vi "GetValue.vi"(8 "error in":errorcluster, 11 "CustomElement in":refnum<class "CustomElement.lvclass">) -> (0 "error out":errorcluster, 2 "Value":string, 3 "CustomElement out":refnum<class "CustomElement.lvclass">)   [LabVIEW 2021, in "ProligentXMLGenerator.lvlib" / "CustomElement.lvclass"]
doc: "This value need to be formated as a valid XML element."
uses:
  CustomElement.lvclass
  CustomElement.lvclass/CustomElement.ctl
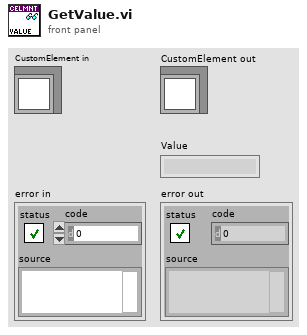
[diagram p1: front panel]
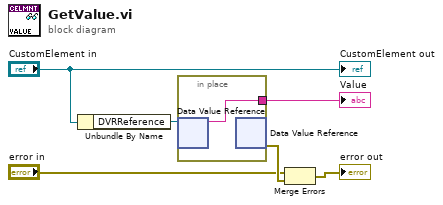
[diagram p0: block diagram]
diagram:
  n1 = Unbundle By Name("CustomElement in") -> ("DVRReference"=w1:refnum<data-value>)
  n2 = in-place "In Place Element Structure" {
    in-place-border: [w7] -> w5
    n3 = in-place-dvr #1(w1) -> (w7:string)  [unwired: 1 out]
    n4 = in-place-dvr #1() -> (w6:errorcluster)  [unwired: 1 in, 1 out]
  }
  "Value" <- w5
  n5 = Merge Errors("error in", w6) -> (→"error out":errorcluster)
  "CustomElement out" <- "CustomElement in"
